vi "tm487_lut.vi"() -> ()   [LabVIEW 2011]
panel:
  in  "out max":i32=255
  in  "in max":i32=65535
  in  "in min":i32
  in  "out min":i32
  out "Timestamp":dbl
  out "DCAM Version":string
  out "Library Version":string
  out "Image":u16[][](graph)
  out "Frames Per Second":dbl
  in  "Quit":bool
  out "Error Out":errorcluster {"code" format="%.0x"}
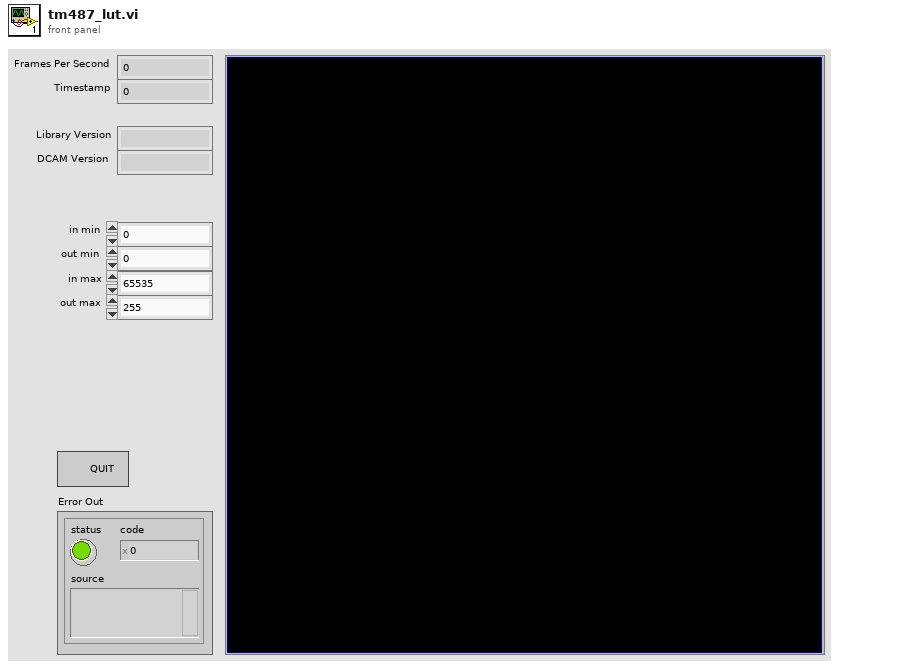
[diagram p1: front panel]
types:
  T1 = cluster{"Capture Library":string, "DCAM-API":string}
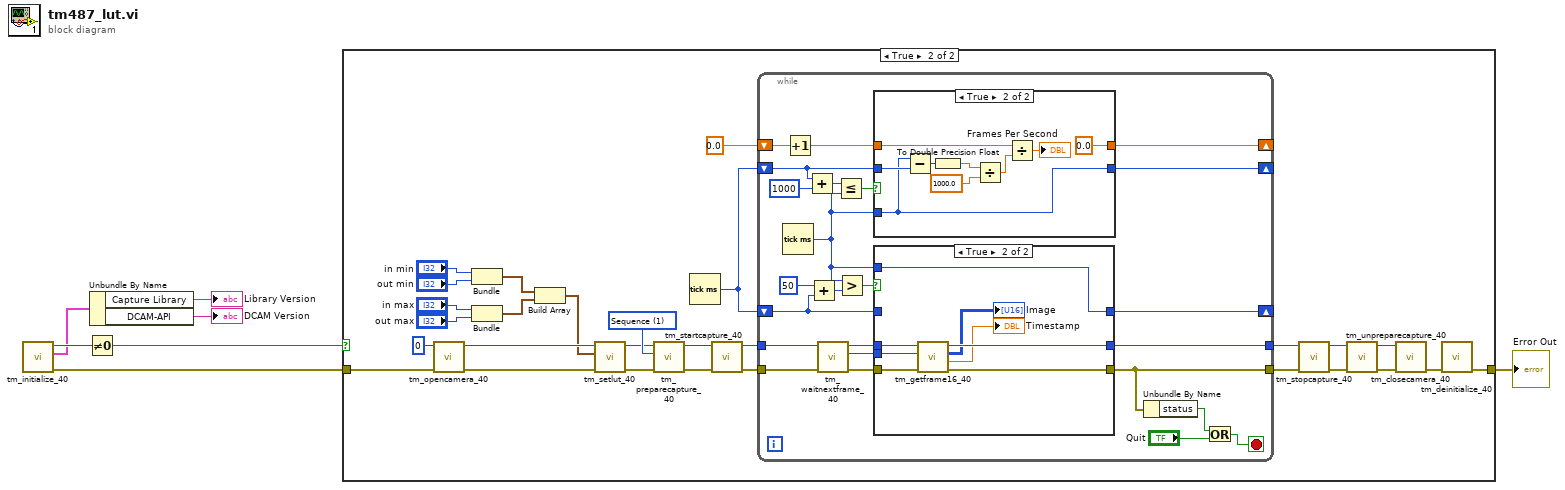
[diagram p0: block diagram]
diagram:
  n1 = call <userlib>:"tm_initialize_40.vi"() -> ("error out"=w4:errorcluster, "Version Info"=w3:T1, "Number Of Cameras"=w5:u32)  [unwired: 8 in, 1 out]
  n2 = Not Equal To 0?(x=w5) -> (x != 0?=w7:bool)
  n3 = Unbundle By Name(w3) -> ("Capture Library"=→"Library Version":string, "DCAM-API"=→"DCAM Version":string)
  n4 = case shown="True" w7 {
    tunnel: w4 -> [w8 w36]
    tunnel: [w8 w33] -> w6
    frame False {
    }
    frame True {
      w24 = 1 items=["Snap", "Sequence"] ("Capture mode")
      n5 = call <userlib>:"tm_opencamera_40.vi"("error in (no error)"=w36, "Camera Index"=u32 0) -> ("error out"=w18:errorcluster, "Handle out"=w19:u32)  [unwired: 7 in, 1 out]
      n6 = Bundle("in min"="in min", "out min"="out min") -> (w9:cluster{"in min":i32, "out min":i32})  [unwired: 1 in]
      n7 = Bundle("in max"="in max", "out max"="out max") -> (w10:cluster{"in max":i32, "out max":i32})  [unwired: 1 in]
      n8 = Build Array(w9, w10) -> (w15:cluster{"in max":i32, "out max":i32}[])
      n9 = call <userlib>:"tm_setlut_40.vi"("error in (no error)"=w18, "LUT Points"=w15, "Handle in"=w19) -> ("error out"=w17:errorcluster, "Handle out"=w16:u32)  [unwired: 7 in]
      n10 = call <userlib>:"tm_preparecapture_40.vi"("error in (no error)"=w17, "Capture mode"=w24, "Handle in"=w16) -> ("error out"=w22:errorcluster, "Handle out"=w23:u32)  [unwired: 5 in, 2 out]
      n11 = Tick Count (ms)() -> (millisecond timer value=w20:u32)
      n12 = call <userlib>:"tm_startcapture_40.vi"("error in (no error)"=w22, "Handle in"=w23) -> ("error out"=w25:errorcluster, "Handle out"=w26:u32)  [unwired: 8 in]
      n13 = while {
        tunnel: [w39] -> w29
        tunnel: [w40] -> w30
        tunnel: w26 -> [w57]
        tunnel: w25 -> [w58]
        shift-right: [w55] -> _
        shift-left: w20 -> [w52]
        shift-right: [w56] -> _
        shift-left: 0.0 -> [w49]
        shift-right: [w38] -> _
        shift-left: w20 -> [w41]
        stop <- w37 stop-if-true
        n14 = Tick Count (ms)() -> (millisecond timer value=w42:u32)
        n15 = Increment(x=w49) -> (x+1=w50:dbl)
        n16 = Add(x=w52, y=u32 1000) -> (x+y=w54:u32)
        n17 = Add(x=u32 50, y=w41) -> (x+y=w44:u32)
        n18 = call <userlib>:"tm_waitnextframe_40.vi"("error in (no error)"=w58, "Handle in"=w57) -> ("error out"=w47:errorcluster, "Frame Index"=w46:i32, "Handle out"=w48:u32)  [unwired: 6 in, 1 out]
        n19 = Less Or Equal?(x=w54, y=w42) -> (x <= y?=w51:bool)
        n20 = Greater?(x=w42, y=w44) -> (0:w43:bool)
        n21 = case shown="True" w51 {
          tunnel: w52 -> [w73 w76]
          tunnel: [w73 w74] -> w55
          tunnel: w50 -> [w72 w80]
          tunnel: w42 -> [_ w74]
          tunnel: [w72 0.0] -> w56
          frame False {
          }
          frame True {
            n22 = Subtract(x=w74, y=w76) -> (x-y=w75:u32)
            n23 = To Double Precision Float(number=w75) -> (double precision float=w82:dbl)
            n24 = Divide(x=w82, y=1000.0) -> (x/y=w79:dbl)
            n25 = Divide(x=w80, y=w79) -> (x/y=→"Frames Per Second":dbl)
          }
        }
        n26 = case shown="True" w43 {
          tunnel: w48 -> [w63 w71]
          tunnel: w47 -> [w62 w70]
          tunnel: w46 -> [_ w64]
          tunnel: w41 -> [w61 _]
          tunnel: w42 -> [_ w69]
          tunnel: [w63 w67] -> w39
          tunnel: [w62 w68] -> w40
          tunnel: [w61 w69] -> w38
          frame False {
          }
          frame True {
            n27 = call <userlib>:"tm_getframe16_40.vi"("error in (no error)"=w70, "Frame Index"=w64, "Handle in"=w71) -> ("error out"=w68:errorcluster, "Timestamp"=→"Timestamp":dbl, "Data"=→"Image":u16[][], "Handle out"=w67:u32)  [unwired: 5 in]
          }
        }
        n28 = Unbundle By Name(w40) -> ("status"=w60:bool)
        n29 = Or(x=w60, y="Quit") -> (x .or. y?=w37:bool)
      }
      n30 = call <userlib>:"tm_stopcapture_40.vi"("error in (no error)"=w30, "Handle in"=w29) -> ("error out"=w27:errorcluster, "Handle out"=w28:u32)  [unwired: 8 in]
      n31 = call <userlib>:"tm_unpreparecapture_40.vi"("error in (no error)"=w27, "Handle in"=w28) -> ("error out"=w32:errorcluster, "Handle out"=w31:u32)  [unwired: 8 in]
      n32 = call <userlib>:"tm_closecamera_40.vi"("error in (no error)"=w32, "Handle in"=w31) -> ("error out"=w34:errorcluster)  [unwired: 9 in]
      n33 = call <userlib>:"tm_deinitialize_40.vi"("error in (no error)"=w34) -> ("error out"=w33:errorcluster)  [unwired: 10 in]
    }
  }
  "Error Out" <- w6
